vi "RSZVB Query Frequency Range.vi"(8 "error in (no error)":errorcluster {"code" format="%.0x"}, 11 "VISA session":refnum<visa-resource-name>) -> (0 "error out":errorcluster {"code" format="%.0x"}, 1 "Maximum Frequency":dbl format="%^.3e", 2 "Minimum Frequency":dbl format="%^.3e", 3 "dup VISA session":refnum<visa-resource-name>)   [LabVIEW 2011]
doc: "Queries the minimum and maximum frequency of the network analyzer.\n\nRemote-control command(s):\nSYSTem:FREQuency? MINimum | MAXimum"
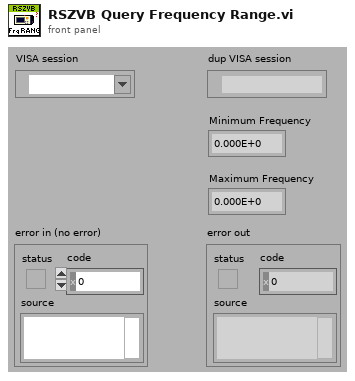
[diagram p1: front panel]
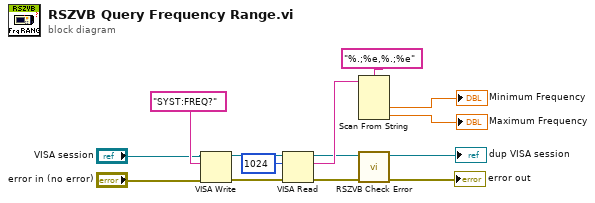
[diagram p0: block diagram]
diagram:
  n1 = VISA Write(VISA resource name="VISA session", write buffer="SYST:FREQ?", error in (no error)="error in (no error)") -> (VISA resource name out=w12:refnum<visa-resource-name>, error out=w13:errorcluster)  [unwired: 1 out]
  n2 = VISA Read(VISA resource name=w12, byte count=u32 1024, error in (no error)=w13) -> (VISA resource name out=w7:refnum<visa-resource-name>, read buffer=w9:string, error out=w8:errorcluster)  [unwired: 1 out]
  n3 = Scan From String(format string="%.;%e,%.;%e", input string=w9) -> (output 1=→"Minimum Frequency":dbl, output 2=→"Maximum Frequency":dbl)  [unwired: 4 in, 3 out]
  n4 = call "RSZVB Check Error.vi"("error in (no error)"=w8, "VISA session"=w7) -> ("error out"=→"error out":errorcluster, "dup VISA session"=→"dup VISA session":refnum<visa-resource-name>)  [unwired: 8 in]
